vi "Get Label Settings for RT.vi"(8 "error in":errorcluster, 11 "label ref in":T1 format="%.0x") -> (0 "error out":errorcluster, 2 "label settings for RT":T2 {"Label Timestamp Channel Data Reference" format="%x"; "Word Initial Raw Value" format="%032.0f"; "Label Disable/Trigger Channel Reference" format="%.0x"; "parameter driver data"."Tx parameter refs" format="%.0x"; "parameter driver data"."Rx block data refs"."Data Reference" format="%.0x"; "SDI" format="%02b"; "label" format="%.0o"}, 3 "Item Ref out":T1 format="%.0x")   [LabVIEW 2020, in "Ballard ARINC 429 Shared.lvlib"]
uses:
  Ballard ARINC 429 Shared.lvlib
  <vilib>/NI VeriStand/Custom Device API/Custom Device API.lvlib
  <vilib>/NI VeriStand/Custom Device API/Get Item Property (U32).vi
  <vilib>/NI VeriStand/Custom Device API/Get Item Property (String).vi
  <vilib>/NI VeriStand/Custom Device API/Get Item Property (U16).vi
  <vilib>/NI VeriStand/Custom Device API/Get Item Property (Boolean).vi
  Custom Device Support/Scripting/Constants.vi
  Custom Device Support/Scripting/Communication Bus Template Scripting.lvlib
  Transfer Type.ctl
  <vilib>/NI VeriStand/Custom Device API/Custom Device Item Ref.ctl
  <vilib>/NI VeriStand/Custom Device API/Data Reference.ctl
  <vilib>/NI VeriStand/Custom Device API/Block Data Reference.ctl
  Encoding and Decoding/Encoding.ctl
  Encoding and Decoding/Encoding and Decoding.lvlib
  Protocol/Implementations/ARINC429/Parameter Definition.ctl
  Protocol/Implementations/ARINC429/ARINC 429.lvclass
  RT Parameters.ctl
  Label.ctl
  RT Label Settings.ctl
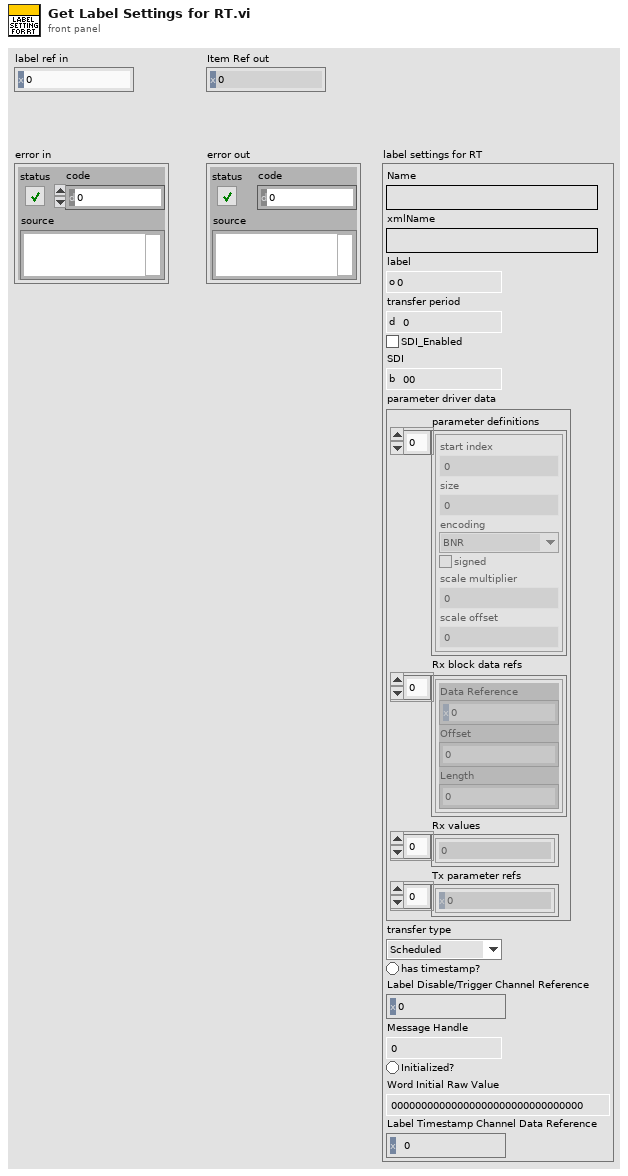
[diagram p1: front panel]
types:
  T1 = typedef "Custom Device API.lvlib/Custom Device Item Ref.ctl" = u64
  T2 = typedef "Ballard ARINC 429 Shared.lvlib/RT Label Settings.ctl" = cluster{"Name":string, "xmlName":string, "label":T3, "transfer period":u32, "SDI_Enabled":bool, "SDI":u8, "parameter driver data":T4, "transfer type":T9, "has timestamp?":bool, "Label Disable/Trigger Channel Reference":T1, "Message Handle":u64, "Initialized?":bool, "Word Initial Raw Value":u32, "Label Timestamp Channel Data Reference":T8}
  T3 = typedef "Ballard ARINC 429 Shared.lvlib/Label.ctl" = u8
  T4 = typedef "Ballard ARINC 429 Shared.lvlib/RT Parameters.ctl" = cluster{"parameter definitions":T5[], "Rx block data refs":T7[], "Rx values":dbl[], "Tx parameter refs":T1[]}
  T5 = typedef "ARINC 429.lvclass/Parameter Definition.ctl" = cluster{"start index":i32, "size":i32, "encoding":T6, "signed":bool, "scale multiplier":dbl, "scale offset":dbl}
  T6 = typedef "Encoding and Decoding.lvlib/Encoding.ctl" = enum16{"BNR", "BCD", "Discrete"}
  T7 = typedef "Custom Device API.lvlib/Block Data Reference.ctl" = cluster{"Data Reference":T8, "Offset":u64, "Length":u64}
  T8 = typedef "Custom Device API.lvlib/Data Reference.ctl" = i32
  T9 = typedef "Ballard ARINC 429 Shared.lvlib/Transfer Type.ctl" = enum16{"Scheduled", "Acyclic", "Block", "Strobe"}
  T10 = typedef "Custom Device API.lvlib/Custom Device Item Info.ctl" = cluster{"Name":string, "Is Channel":bool, "GUID":string, "Is Waveform":bool}
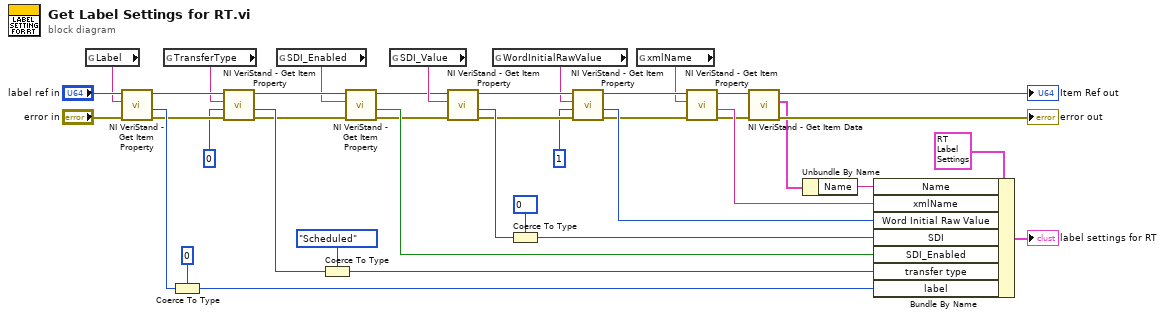
[diagram p0: block diagram]
diagram:
  n1 = global read "Constants.vi" "Label"() -> (w6:string)
  n2 = call-poly <vilib>:"NI VeriStand - Get Item Property.vi"("error in (no error)"="error in", "Property Name"=w6, "Item Ref in"="label ref in") -> ("error out"=w14:errorcluster, "Value"=w35:u32, "Item Ref out"=w13:T1)  [unwired: 5 in, 1 out]
  n3 = global read "Constants.vi" "TransferType"() -> (w12:string)
  n4 = Coerce To Type(0:w35, 1:T3 0 ("label")) -> (2:w36:T3)
  n5 = call-poly <vilib>:"NI VeriStand - Get Item Property.vi"("error in (no error)"=w14, "Default Value"=u16 0, "Property Name"=w12, "Item Ref in"=w13) -> ("error out"=w15:errorcluster, "Value"=w32:u16, "Item Ref out"=w16:T1)  [unwired: 4 in, 1 out]
  n6 = global read "Constants.vi" "SDI_Enabled"() -> (w9:string)
  n7 = Coerce To Type(0:w32, 1:Transfer_Type."Scheduled" ("transfer type")) -> (2:w33:T9)
  n8 = call-poly <vilib>:"NI VeriStand - Get Item Property.vi"("error in (no error)"=w15, "Property Name"=w9, "Item Ref in"=w16) -> ("error out"=w5:errorcluster, "Value"=w30:bool, "Item Ref out"=w4:T1)  [unwired: 5 in, 1 out]
  n9 = global read "Constants.vi" "SDI_Value"() -> (w10:string)
  n10 = call-poly <vilib>:"NI VeriStand - Get Item Property.vi"("error in (no error)"=w5, "Property Name"=w10, "Item Ref in"=w4) -> ("error out"=w19:errorcluster, "Value"=w28:u32, "Item Ref out"=w18:T1)  [unwired: 5 in, 1 out]
  n11 = global read "Constants.vi" "WordInitialRawValue"() -> (w17:string)
  n12 = Coerce To Type(0:w28, 1:u8 0 ("SDI")) -> (2:w29:u8)
  n13 = call-poly <vilib>:"NI VeriStand - Get Item Property.vi"("error in (no error)"=w19, "Default Value"=u32 1, "Property Name"=w17, "Item Ref in"=w18) -> ("error out"=w23:errorcluster, "Value"=w26:u32, "Item Ref out"=w20:T1)  [unwired: 4 in, 1 out]
  n14 = global read "Constants.vi" "xmlName"() -> (w11:string)
  n15 = call-poly <vilib>:"NI VeriStand - Get Item Property.vi"("error in (no error)"=w23, "Property Name"=w11, "Item Ref in"=w20) -> ("error out"=w22:errorcluster, "Value"=w37:string, "Item Ref out"=w21:T1)  [unwired: 5 in, 1 out]
  n16 = call <vilib>:"NI VeriStand - Get Item Data.vi"("error in (no error)"=w22, "Item Ref in"=w21) -> ("error out"=→"error out":errorcluster, "Item Info"=w2:T10, "Item Ref out"=→"Item Ref out":T1)  [unwired: 6 in, 1 out]
  n17 = Unbundle By Name(w2) -> ("Name"=w25:string)
  n18 = Bundle By Name(cluster=T2 {"Name"="", "xmlName"="", "label"=0, "transfer period"=0, "SDI_Enabled"=FALSE, "SDI"=0, "parameter driver data"={"parameter definitions"=[], "Rx block data refs"=[], "Rx values"=[], "Tx parameter refs"=[]}, "transfer type"=enum."Scheduled", "has timestamp?"=FALSE, "Label Disable/Trigger Channel Reference"=0, "Message Handle"=0, "Initialized?"=FALSE, "Word Initial Raw Value"=0, "Label Timestamp Channel Data Reference"=0} ("label settings for RT"), "Name"=w25, "xmlName"=w37, "Word Initial Raw Value"=w26, "SDI"=w29, "SDI_Enabled"=w30, "transfer type"=w33, "label"=w36) -> (→"label settings for RT":T2)
